vi "Update_Extrapol_Results.vi"(8 "error in (no error)":errorcluster, 9 "results string":string, 10 "PlotID":string, 11 "Analysis in":refnum<class "Analysis.lvclass">) -> (0 "error out":errorcluster, 3 "Analysis out":refnum<class "Analysis.lvclass">)   [LabVIEW 2017]
doc: "Updates the Extrapolation Results Table of the AnalysisObject with the given data from the PlotID (whic stroes the isotope name)"
uses:
  MSControl/Classes/Analysis/Analysis.lvclass
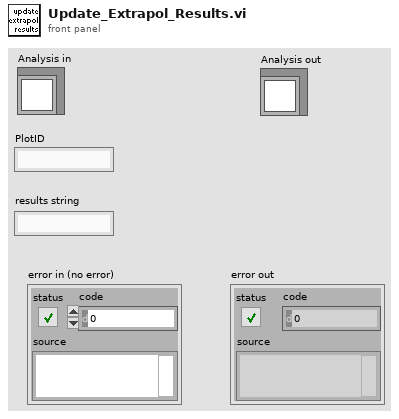
[diagram p1: front panel]
types:
  T1 = typedef "ExtrapolationResultsArray.ctl" = string[][]
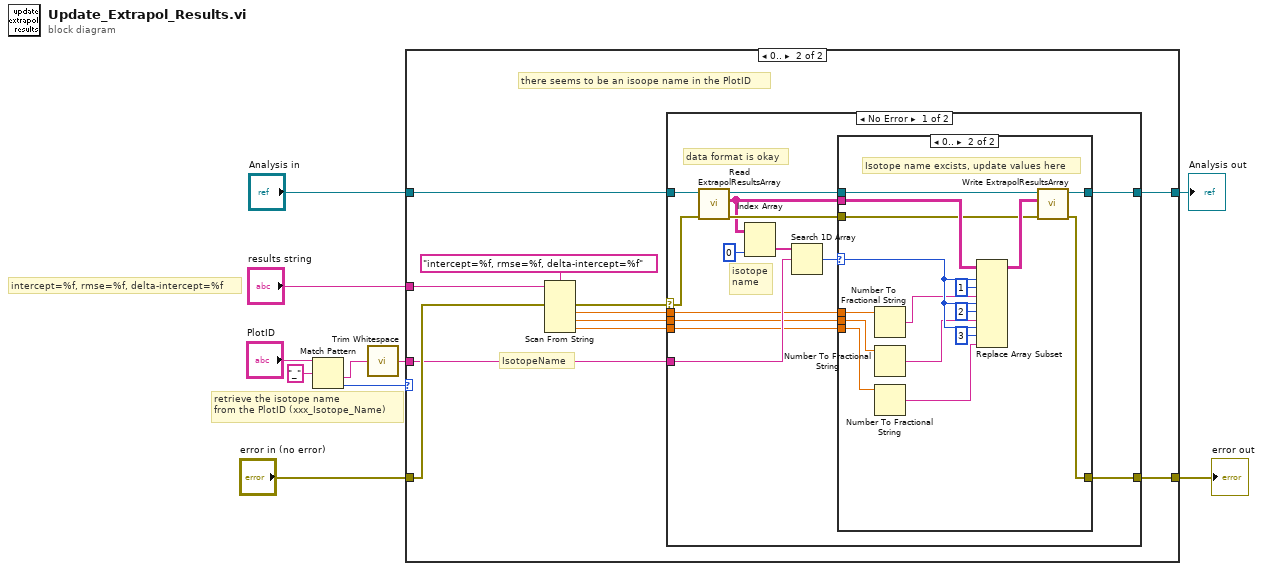
[diagram p0: block diagram]
diagram:
  # "intercept=%f, rmse=%f, delta-intercept=%f"
  # "retrieve the isotope name\nfrom the PlotID (xxx_Isotope_Name)"
  n1 = Match Pattern(string="PlotID", regular expression="_") -> (after substring=w5:string, offset past match=w9:i32)  [unwired: 1 in, 2 out]
  n2 = call <vilib>:"Trim Whitespace.vi"("string"=w5) -> ("trimmed string"=w4:string)  [unwired: 1 in]
  n3 = case shown="0.." w9 {
    tunnel: "Analysis in" -> [w11 w20]
    tunnel: "results string" -> [_ w23]
    tunnel: w4 -> [_ w14]
    tunnel: "error in (no error)" -> [w12 w16]
    tunnel: [w12 w15] -> w2
    tunnel: [w11 w13] -> w1
    frame -1, Default {
      # "no isotope name found"
    }
    frame 0.. {
      # "IsotopeName"
      # "there seems to be an isoope name in the PlotID"
      n4 = Scan From String(format string="intercept=%f, rmse=%f, delta-intercept=%f", input string=w23, error in=w16) -> (error out=w21:errorcluster, output 1=w19:dbl, output 2=w18:dbl, output 3=w17:dbl)  [unwired: 4 in, 2 out]
      n5 = case shown="No Error" w21 {
        selector: w21 -> [w36 w57]
        tunnel: w20 -> [w37 w56]
        tunnel: w19 -> [w28 _]
        tunnel: w18 -> [w27 _]
        tunnel: w17 -> [w26 _]
        tunnel: [w30 w57] -> w15
        tunnel: w14 -> [w33 _]
        tunnel: [w24 w56] -> w13
        frame No Error {
          # "isotope\nname"
          # "data format is okay"
          n6 = call-dynamic "Read ExtrapolResultsArray.vi"("error in (no error)"=w36, "Analysis in"=w37) -> ("error out"=w31:errorcluster, "ExtrapolResultsArray"=w29:T1, "Analysis out"=w25:refnum<class "Analysis.lvclass">)  [unwired: 7 in]
          n7 = Index Array(array=w29, index (col)=0 ("disabled index (col)")) -> (element=w34:string[])  [unwired: 1 in]
          n8 = Search 1D Array(1D array=w34, element=w33) -> (index of element=w32:i32)  [unwired: 1 in]
          n9 = case shown="0.." w32 {
            selector: w32 -> [_ w52]
            tunnel: w31 -> [w39 w48]
            tunnel: [w39 w47] -> w30
            tunnel: w29 -> [_ w55]
            tunnel: w28 -> [_ w45]
            tunnel: w27 -> [_ w44]
            tunnel: w26 -> [_ w43]
            tunnel: w25 -> [w38 w50]
            tunnel: [w38 w46] -> w24
            frame -1, Default {
              # "isotope name doesn't excist\nin the extrapolation table"
            }
            frame 0.. {
              # "Isotope name excists, update values here"
              n10 = Number To Fractional String(number=w45) -> (F-format string=w42:string)  [unwired: 3 in]
              n11 = Number To Fractional String(number=w44) -> (F-format string=w41:string)  [unwired: 3 in]
              n12 = Number To Fractional String(number=w43) -> (F-format string=w40:string)  [unwired: 3 in]
              n13 = Replace Array Subset(array=w55, new element #1=w42, index (row) #1=w52, index (col) #1=1 ("disabled index (col)"), new element #2=w41, index (row) #2=w52, index (col) #2=2 ("disabled index (col)"), new element #3=w40, index (row) #3=w52, index (col) #3=3 ("disabled index (col)")) -> (w49:T1)
              n14 = call-dynamic "Write ExtrapolResultsArray.vi"("error in (no error)"=w48, "ExtrapolResultsArray"=w49, "Analysis in"=w50) -> ("error out"=w47:errorcluster, "Analysis out"=w46:refnum<class "Analysis.lvclass">)  [unwired: 7 in]
            }
          }
        }
        frame Error {
          # "someting is wrong with the data format"
        }
      }
    }
  }
  "error out" <- w2
  "Analysis out" <- w1
